vi "Plot add row.vi"(8 "error in (no error)":errorcluster, 11 "Refs":T1) -> (0 "error out":errorcluster)   [LabVIEW 2021, in "RocketPlot.lvlib"]
uses:
  RocketPlot.lvlib
  TypeDefs/Plot UI references.ctl
  Classes/RocketPlotHandle/RocketPlotHandle.lvclass
  <userlib>/bjustice/TipStripOOPanel/Classes/TipPanelHandle/TipPanelHandle.lvclass
  TypeDefs/Plot top row.ctl
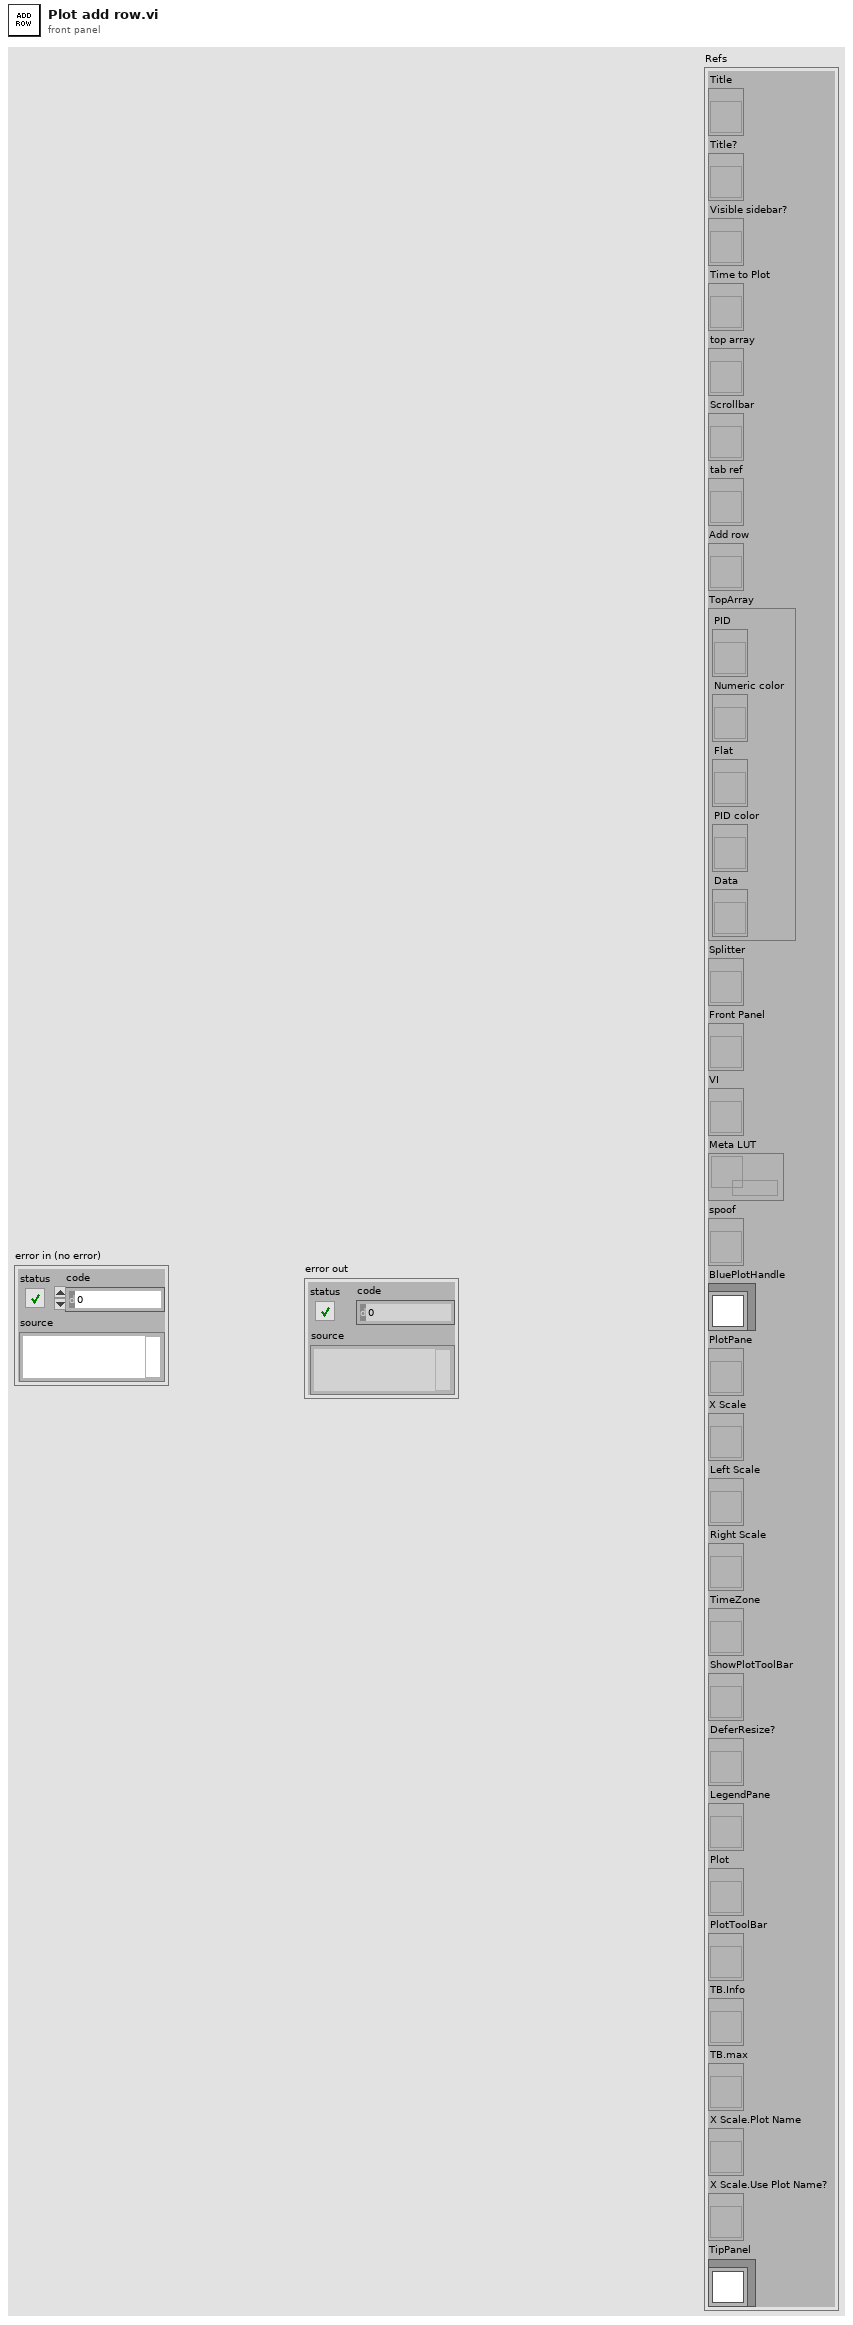
[diagram p1: front panel]
types:
  T1 = typedef "RocketPlot.lvlib/Plot UI references.ctl" = cluster{"Title":refnum<vi>, "Title?":refnum<vi>, "Visible sidebar?":refnum<vi>, "Time to Plot":refnum<vi>, "top array":refnum<vi>, "Scrollbar":refnum<vi>, "tab ref":refnum<vi>, "Add row":refnum<vi>, "TopArray":cluster{"PID":refnum<vi>, "Numeric color":refnum<vi>, "Flat":refnum<vi>, "PID color":refnum<vi>, "Data":refnum<vi>}, "Splitter":refnum<vi>, "Front Panel":refnum<vi>, "VI":refnum<vi>, "Meta LUT":refnum<data-value>, "spoof":refnum<vi>, "BluePlotHandle":refnum<class "RocketPlotHandle.lvclass">, "PlotPane":refnum<vi>, "X Scale":refnum<vi>, "Left Scale":refnum<vi>, "Right Scale":refnum<vi>, "TimeZone":refnum<vi>, "ShowPlotToolBar":refnum<vi>, "DeferResize?":refnum<vi>, "LegendPane":refnum<vi>, "Plot":refnum<vi>, "PlotToolBar":refnum<vi>, "TB.Info":refnum<vi>, "TB.max":refnum<vi>, "X Scale.Plot Name":refnum<vi>, "X Scale.Use Plot Name?":refnum<vi>, "TipPanel":refnum<class "TipPanelHandle.lvclass">}
  T2 = typedef "Plot top row.ctl" = cluster{"PID":string, "index":i32, "PID color":u32, "right axis?":bool, "Flatline?":bool, "Numeric color":u32, "Data":string, "Flat":string}
  T3 = typedef "RocketPlot.lvlib/Plot top row.ctl" = cluster{"PID":string, "index":i32, "PID color":u32, "right axis?":bool, "Flatline?":bool, "Numeric color":u32, "Data":string, "Flat":string}
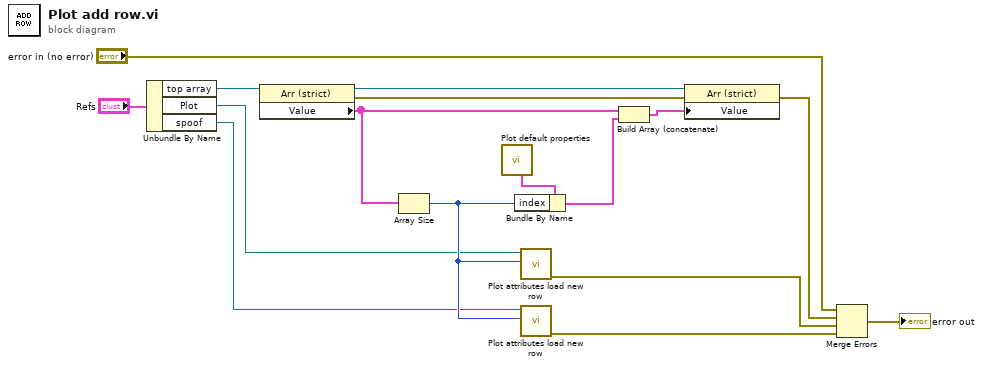
[diagram p0: block diagram]
diagram:
  n1 = Unbundle By Name("Refs") -> ("top array"=w3:refnum<vi>, "Plot"=w2:refnum<vi>, "spoof"=w1:refnum<vi>)
  n2 = property class="Arr (strict)"(reference=w3) -> (reference out=w16:refnum<vi>, error out=w12:errorcluster, "Value"=w15:T2[])  [unwired: 1 in]
  n3 = Array Size(array=w15) -> (size(s)=w8:i32)
  n4 = call "Plot default properties.vi"() -> ("Default plot UI"=w5:T3)  [unwired: 7 in, 4 out]
  n5 = Bundle By Name(cluster=w5, "index"=w8) -> (w14:T3)
  n6 = call "Plot attributes load new row.vi"("Plot Index"=w8, "Plot"=w2) -> ("error out"=w7:errorcluster)  [unwired: 8 in, 1 out]
  n7 = call "Plot attributes load new row.vi"("Plot Index"=w8, "Plot"=w1) -> ("error out"=w6:errorcluster)  [unwired: 8 in, 1 out]
  n8 = Build Array (concatenate)(w15, w14) -> (w13:T3[])
  n9 = property class="Arr (strict)"(reference=w16, error in=w12, "Value"=w13) -> (error out=w11:errorcluster)  [unwired: 1 out]
  n10 = Merge Errors("error in (no error)", w11, w7, w6) -> (→"error out":errorcluster)
